vi "Adaptive FF.vi"(5 "Reset":bool=TRUE, 8 "input valid":bool=TRUE, 10 "Disable e(n)":bool) -> (0 "output valid":bool, 3 "done":bool)   [LabVIEW 2018]
uses:
  <vilib>/rvi/Emulation/niFpgaEmulationIsFPGAContextNoSignature.vi
  <vilib>/rvi/DataTransferAndStorage/Container/Common/niFpgaContainerGetUniqueNameForEmu.vi
  <vilib>/rvi/Memory/Memory_Emulation/niFpgaMemoryEmulationCacheClearOnFirstRun.vi
  <vilib>/rvi/Memory/Memory_Emulation/nirvimemoryEmulationManagerCache_MakeExclusive.vi
  <vilib>/rvi/Memory/Memory_Emulation/niFpgaMemoryEmulationValidateCache.vi
  <vilib>/rvi/Memory/Memory_Emulation/nirvimemoryEmulationManagerCache_InsertValue.vi
  <vilib>/Utility/error.llb/Clear Errors.vi
  <vilib>/rvi/Memory/Memory_Emulation/nirvimemoryEmulationManagerCache_ReleaseExclusive.vi
  <vilib>/rvi/Memory/Memory_Emulation/nirvimemoryEmulationManagerCache_GetValue.vi
  <vilib>/rvi/Memory/Memory_Emulation/nirvimemoryEmulationManagerCache_SetValue.vi
  <vilib>/rvi/Emulation/niFpgaProcessEmulError.vi
  <vilib>/rvi/Emulation/niFpgaSctlEmulationGetInTimedLoop.vi
  <instrlib>/_niInstr/Basic Elements/v1/FPGA/Private/Count Down U32.vi
  <vilib>/rvi/DataTransferAndStorage/Container/XNode/niFpgaContainer.xnode
  <vilib>/rvi/DataTransferAndStorage/Register/Emulation/niFpgaRegisterEmulation.vi
  <instrlib>/_niInstr/Basic Elements/v1/FPGA/niInstr Basic Elements v1 FPGA.lvlib
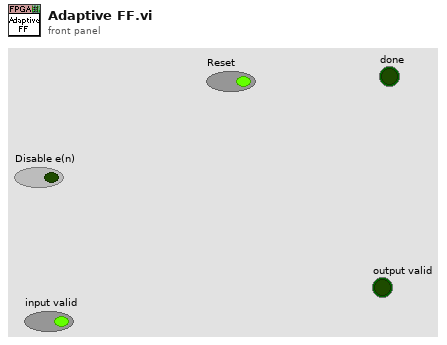
[diagram p1: front panel]
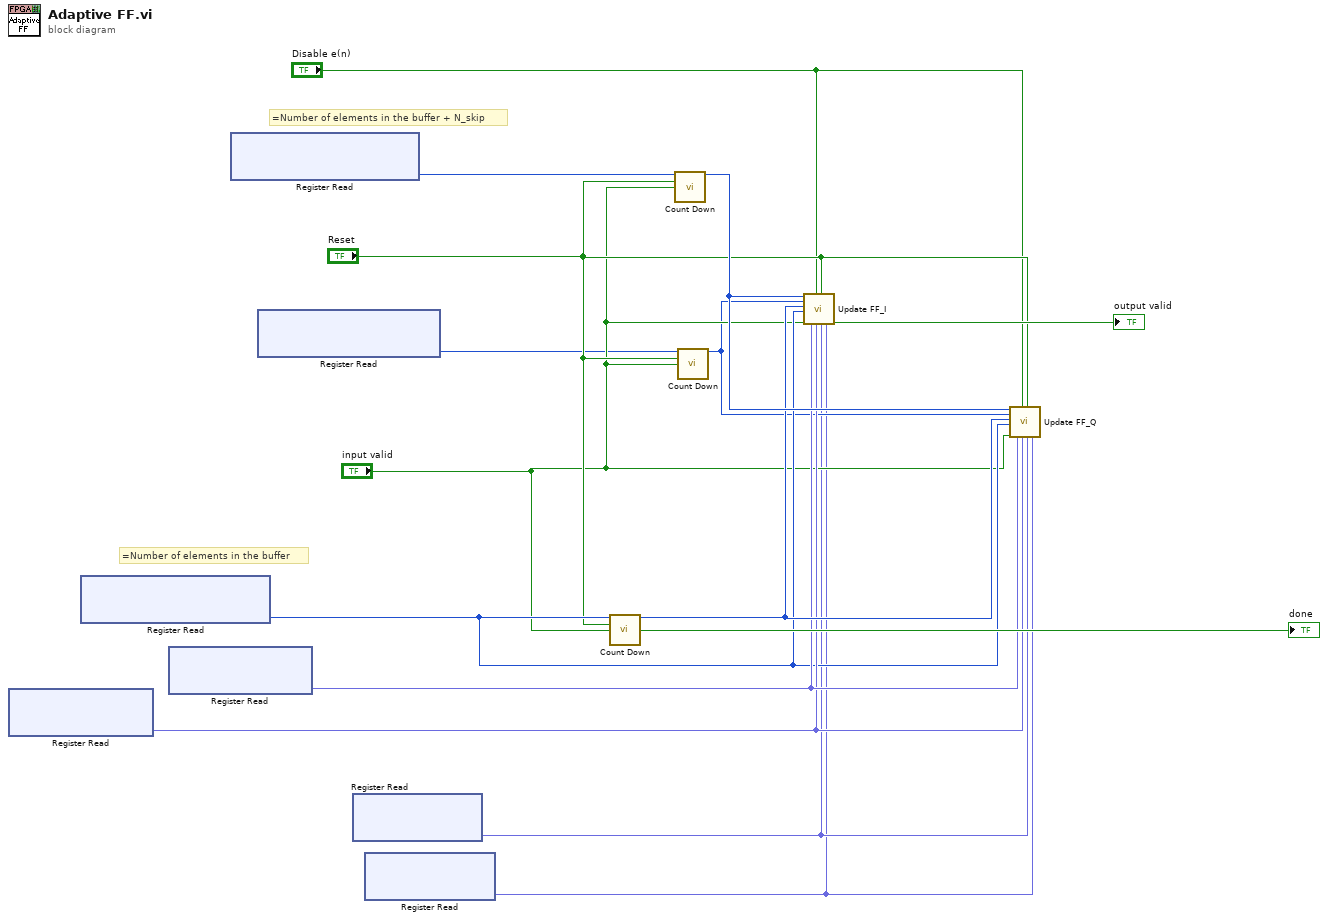
[diagram p0: block diagram]
diagram:
  # "=Number of elements in the buffer"
  # "=Number of elements in the buffer + N_skip"
  n1 = xnode ("Register Read")() -> ("Data"=w10:fxp<+/-,32,2>)  [unwired: 1 in, 1 out]
  n2 = xnode ("Register Read")() -> ("Data"=w9:u32)  [unwired: 1 in, 1 out]
  n3 = xnode ("Register Read")() -> ("Data"=w11:fxp<+/-,32,2>)  [unwired: 1 in, 1 out]
  n4 = xnode ("Register Read")() -> ("Data"=w8:u32)  [unwired: 1 in, 1 out]
  n5 = xnode "Register Read"() -> ("Data"=w5:u32)  [unwired: 1 in, 1 out]
  n6 = xnode "Register Read"() -> ("Data"=w2:fxp<+/-,32,4>)  [unwired: 1 in, 1 out]
  n7 = xnode "Register Read"() -> ("Data"=w1:fxp<+/-,32,17>)  [unwired: 1 in, 1 out]
  n8 = call-poly <instrlib>:"Count Down.vi"("count in"=w9, "load"="Reset", "decrement"="input valid") -> ("count out"=w12:u32, "terminal count"=→"done":bool)  [unwired: 11 in]
  n9 = call-poly <instrlib>:"Count Down.vi"("count in"=w8, "load"="Reset", "decrement"="input valid") -> ("count out"=w13:u32)  [unwired: 11 in, 1 out]
  n10 = call-poly <instrlib>:"Count Down.vi"("count in"=w5, "load"="Reset", "decrement"="input valid") -> ("count out"=w4:u32)  [unwired: 11 in, 1 out]
  n11 = call "Update FF_I.vi"("source adress PID out"=w13, "source adress e(n)"=w4, "destination adress"=w12, "Buffer size"=w9, "input valid"="input valid", "a0"=w11, "Disable e(n)"="Disable e(n)", "b0"=w10, "Reset"="Reset", "cavity filter - a"=w2, "cavity filter - b"=w1) -> ("output valid"=→"output valid":bool)  [unwired: 8 in]
  n12 = call "Update FF_Q.vi"("source adress PID out"=w13, "source adress e(n)"=w4, "destination adress"=w12, "Buffer size"=w9, "input valid"="input valid", "a0"=w11, "Disable e(n)"="Disable e(n)", "b0"=w10, "Reset"="Reset", "cavity filter - a"=w2, "cavity filter - b"=w1) -> ()  [unwired: 8 in, 1 out]
